vi "DSCProgIOCloopBind FP.vi"() -> ()   [LabVIEW 2011]
uses:
  <vilib>/variable/tagger/epicsserver/API/internal/List PVs (By Ref).vi
  <vilib>/variable/tagger/epicsserver/API/internal/Undeploy EPICS Server (By Ref).vi
  <vilib>/variable/tagger/epicsserver/API/internal/EPICSServerClass/EPICSServer.lvclass
  <vilib>/variable/tagger/epicsserver/API/NI_EPICS_Server.lvlib
  <vilib>/lvdsc/NI_DSC.lvlib
  Program Files (x86)/National Instruments/LabVIEW 2011/resource/objmgr/nvio.rc
panel:
  out "data out 3":dbl
  in  "data in":dbl
  out "data out 2":dbl
  out "data out":dbl
  out "PVs":string[](array[string])
  out "error out":errorcluster
  in  "stop":bool
  out "EPICS Server URL out":string
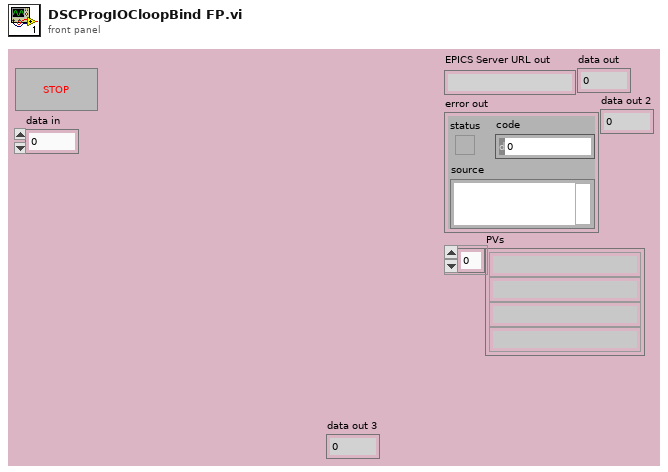
[diagram p1: front panel]
types:
  T1 = enum32{"No PSP", "Read", "Write", "Write & Read"}
  T2 = enum32{"u32BitField", "bool", "double", "string", "int8", "uint8", "int16", "uint16", "int32", "uint32", "int64", "uint64", "single", "double waveform", "int16 waveform", "array of boolean", "array of int8", "array of uint8", "array of int16", "array of uint16", "array of int32", "array of uint32", "array of int64", "array of uint64", "array of single", "array of double", "array of double waveform", "array of int16 waveform", "array of string", "variant", "timestamp", "fixed point", "custom"}
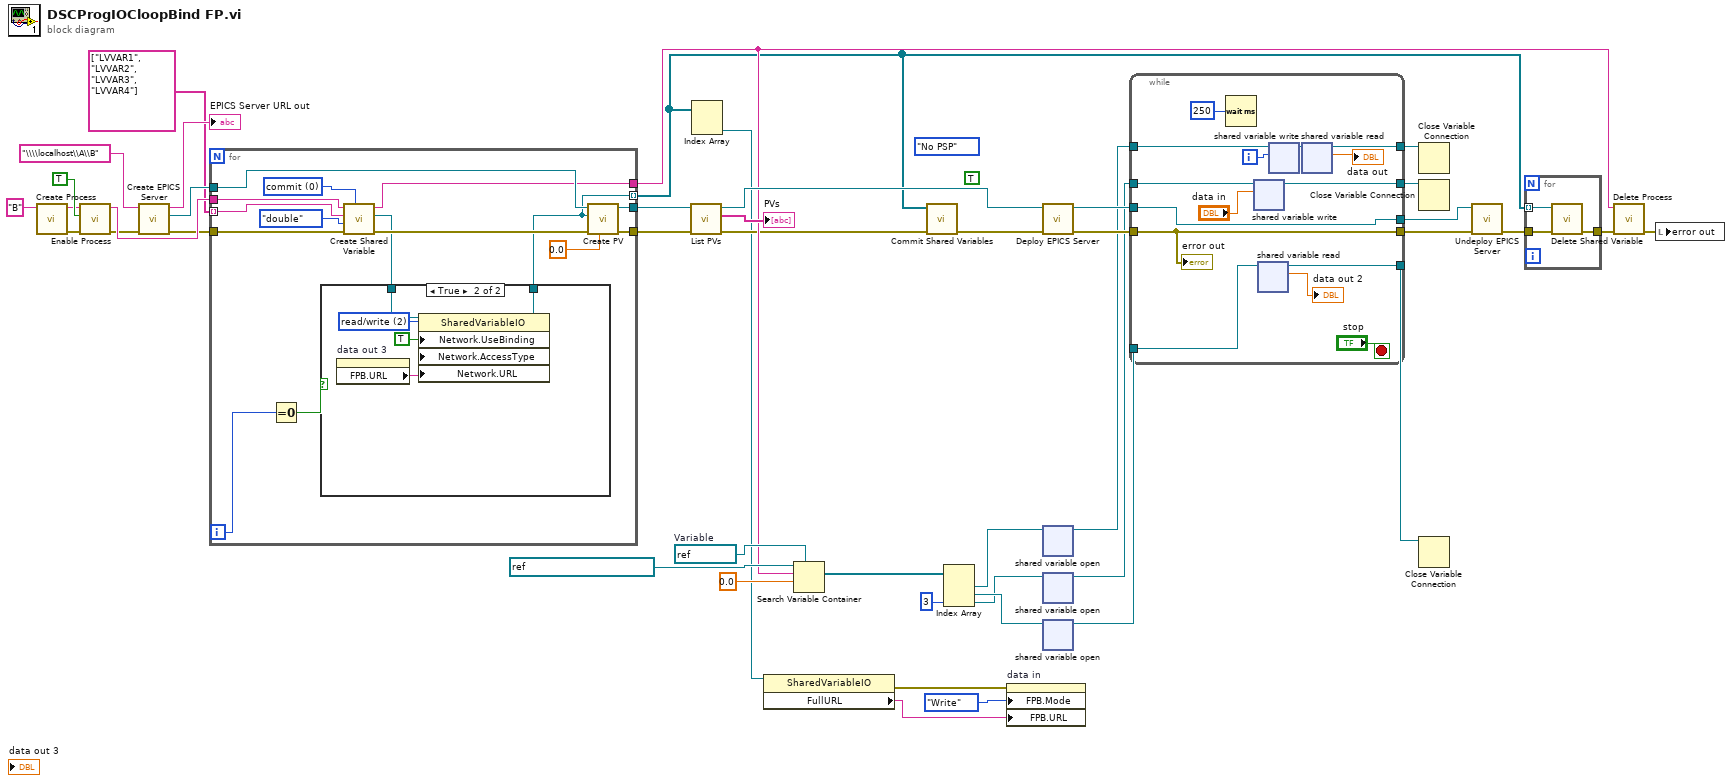
[diagram p0: block diagram]
diagram:
  (unwired) TRUE ("Data Binding:LED Visible")
  (unwired) T1."No PSP" ("Data Binding:Mode")
  w30 = refnum<k21> refnum  # Variable
  n1 = call <vilib>:"Create Process.vi"("process name"="B") -> ("error out"=w24:errorcluster, "process name out"=w20:string)  [unwired: 9 in]
  n2 = call <vilib>:"Enable Process.vi"("error in (no error)"=w24, "run?"=TRUE, "process name"=w20) -> ("error out"=w14:errorcluster, "process name out"=w19:string)  [unwired: 7 in]
  n3 = call <vilib>:"Create EPICS Server.vi"("error in (no error)"=w14, "EPICS Server URL in"="\\\\localhost\\A\\B") -> ("error out"=w13:errorcluster, "EPICS Server ref"=w44:refnum<data-value>, "EPICS Server URL out"=→"EPICS Server URL out":string)  [unwired: 7 in]
  n4 = for {
    tunnel: w44 -> [w59]
    tunnel: [w57] -> w39
    tunnel: [w56] -> w38
    tunnel: [w54] -> w21
    tunnel: w19 -> [w53]
    tunnel: [w47] -> w3 mode=indexing
    tunnel: string[] ["LVVAR1", "LVVAR2", "LVVAR3", "LVVAR4"] -> [w52] mode=indexing
    tunnel: w13 -> [w51]
    i -> [w46]
    w49 = u16 0 items=["commit", "buffer"] ("set mode")
    n5 = Equal To 0?(x=w46) -> (x = 0?=w45:bool)
    n6 = call <vilib>:"Create Shared Variable.vi"("set mode"=w49, "error in (no error)"=w51, "data type"=T2."double", "shared variable name"=w52, "process name"=w53) -> ("error out"=w50:errorcluster, "shared variable"=w48:refnum<k21>, "process name out"=w54:string)  [unwired: 4 in]
    n7 = case shown="True" w45 {
      tunnel: w48 -> [w60 w65]
      tunnel: [w60 w64] -> w47
      frame False {
      }
      frame True {
        w61 = u32 2 items=["read only", "write only", "read/write"] ("Network.AccessType")
        n8 = property on="data out 3" class="DigNum (strict)"() -> ("FPB.URL"=w63:string)  [unwired: 2 in, 2 out]
        n9 = property class="SharedVariableIO"(reference=w65, "Network.UseBinding"=TRUE, "Network.AccessType"=w61, "Network.URL"=w63) -> (reference out=w64:refnum<k21>)  [unwired: 1 in, 1 out]
      }
    }
    n10 = call <vilib>:"Create PV.vi"("data type"=0.0, "error in (no error)"=w50, "variable path"=w47, "EPICS Server ref in"=w59) -> ("error out"=w56:errorcluster, "EPICS Server ref out"=w57:refnum<data-value>)  [unwired: 6 in]
  }
  n11 = call-poly <vilib>:"List PVs.vi"("error in (no error)"=w38, "EPICS Server ref in"=w39) -> ("error out"=w18:errorcluster, "PVs"=→"PVs":string[], "EPICS Server ref out"=w36:refnum<data-value>)  [unwired: 7 in]
  n12 = Index Array(array=w3) -> (element #2=w1:refnum<k21>)  [unwired: 2 in, 1 out]
  n13 = property class="SharedVariableIO"(reference=w1) -> (error out=w5:errorcluster, "FullURL"=w6:string)  [unwired: 1 in, 1 out]
  n14 = Search Variable Container(7:w30, 9:0.0, 10:w21, 11:refnum<k21> "ni.var.psp://localhost/" ("container refnum in")) -> (2:w33:refnum<k21>[])  [unwired: 2 in, 2 out]
  n15 = call <vilib>:"Commit Shared Variables.vi"("error in (no error)"=w18, "shared variables"=w3) -> ("error out"=w28:errorcluster)  [unwired: 8 in, 1 out]
  n16 = Index Array(array=w33, index #3=3 ("index")) -> (element #1=w29:refnum<k21>, element #2=w17:refnum<k21>, element #3=w10:refnum<k21>)  [unwired: 2 in]
  n17 = property on="data in" class="DigNum (strict)"(error in=w5, "FPB.Mode"=T1."Write" ("Data Binding:Mode"), "FPB.URL"=w6) -> ()  [unwired: 1 in, 2 out]
  n18 = call <vilib>:"Deploy EPICS Server.vi"("error in (no error)"=w28, "EPICS Server ref in"=w36) -> ("error out"=w35:errorcluster, "EPICS Server ref out"=w42:refnum<data-value>)  [unwired: 8 in]
  n19 = shared-variable-open(w29) -> (w4:refnum<k21>)  [unwired: 2 in, 1 out]
  n20 = shared-variable-open(w10) -> (w9:refnum<k21>)  [unwired: 2 in, 1 out]
  n21 = shared-variable-open(w17) -> (w2:refnum<k21>)  [unwired: 2 in, 1 out]
  n22 = while {
    tunnel: w42 -> [w79]
    tunnel: [w79] -> w41
    tunnel: [w78] -> w40
    tunnel: w35 -> [w78]
    tunnel: w4 -> [w76]
    tunnel: [w67] -> w31
    tunnel: w2 -> [w74]
    tunnel: [w73] -> w16
    tunnel: w9 -> [w71]
    tunnel: [w70] -> w8
    i -> [w77]
    stop <- "stop" stop-if-true
    n23 = Wait (ms)(milliseconds to wait=u32 250) -> ()  [unwired: 1 out]
    n24 = shared-variable-write(w71, "data in") -> (w70:refnum<k21>)  [unwired: 1 in, 1 out]
    n25 = shared-variable-read(w74) -> (w73:refnum<k21>, →"data out 2":dbl)  [unwired: 1 in, 2 out]
    n26 = shared-variable-write(w76, w77) -> (w68:refnum<k21>)  [unwired: 1 in, 1 out]
    n27 = shared-variable-read(w68) -> (w67:refnum<k21>, →"data out":dbl)  [unwired: 1 in, 2 out]
    "error out" <- w78
  }
  n28 = Close Variable Connection(11:w31) -> ()  [unwired: 1 in, 1 out]
  n29 = Close Variable Connection(11:w8) -> ()  [unwired: 1 in, 1 out]
  n30 = Close Variable Connection(11:w16) -> ()  [unwired: 1 in, 1 out]
  n31 = call-poly <vilib>:"Undeploy EPICS Server.vi"("error in (no error)"=w40, "EPICS Server ref"=w41) -> ("error out"=w34:errorcluster)  [unwired: 9 in]
  n32 = for {
    tunnel: w34 -> [w83]
    tunnel: [w82] -> w27
    tunnel: w3 -> [w81] mode=indexing
    n33 = call <vilib>:"Delete Shared Variable.vi"("error in (no error)"=w83, "shared variable"=w81) -> ("error out"=w82:errorcluster)  [unwired: 9 in]
  }
  n34 = call <vilib>:"Delete Process.vi"("error in (no error)"=w27, "process name"=w21) -> ("error out"=w12:errorcluster)  [unwired: 9 in]
  n35 = local write "error out"(w12) -> ()
